vi "bats.parser.hostToFpga.testRunner.vi"(9 "Test.Messages":variant[](array[variant]), 10 "Expected OrderBook.Command[]":T1[](array[typedef])=[{"type"=enum."AddOrder", "side"=66, "orderId "=3544385890602799695, "quantity"=20000, "symbol"=4702127773838213120, "price"=9050, "executed.qty"=0, "canceled.qty"=0, "remaining.qty"=0, "seconds"=0, "nanoseconds"=447000, "Add"=FALSE, "Edit"=FALSE, "Remove"=FALSE}, {"type"=enum."AddOrder", "side"=67, "orderId "=0, "quantity"=30000, "symbol"=4702127773838213120, "price"=9060, "executed.qty"=0, "canceled.qty"=0, "remaining.qty"=0, "seconds"=0, "nanoseconds"=447000, "Add"=FALSE, "Edit"=FALSE, "Remove"=FALSE}] {"symbol" format="%.0x"; "orderId" format="%.0x"; "side" format="%.0x"}, 11 "Test.MessagesOld":T3[](array[typedef])) -> (0 "Failures.Count":i32=1, 2 "Passed":bool, 3 "OrderBook.Command[]":T1[](array[typedef]) {"symbol" format="%.0x"; "orderId" format="%.0x"; "side" format="%.0x"}, 4 "Debug":u64[](array[numeric]) format="%.0x")   [LabVIEW 2022 SP3]
uses:
  fpga/common/orderbook.command.ctl
  fpga/common/orderbook.command.type.ctl
  Message.Spec.ctl
  pitch/oldMessageType.ctl
  pitch/AddOrder/AddOrderLong.Parameters.ctl
  pitch/Time/Time.Parameters.ctl
  pitch/SequencedUnitHeader/SequencedUnitHeader.Parameters.ctl
  pitch/ModifyOrder/ModifyOrderLong.Parameters.ctl
  <vilib>/rvi/interface/RandomDataEmulation/nirviRandomDataOpen.vi
  <vilib>/rvi/interface/common/niFpgaCacheSessionInfoDynamic.vi
  <vilib>/Utility/error.llb/Error Cluster From Error Code.vi
  <vilib>/rvi/errors/niLvFpgaAdjustHostInterfaceError.vi
  <vilib>/FPGAPlugInAG/Dynamic/niLvFpga_Close_Dynamic.vi
  <vilib>/rvi/interface/nirviOpenFPGA/nirviOpenFPGA.xnode
  fpga/bats.parser/bats.parser.test.vi
  <vilib>/rvi/interface/nirviReadWriteControl/nirviReadWriteControl.xnode
  <vilib>/rvi/interface/nirviMethod/nirviMethod.xnode
  <vilib>/rvi/interface/nirviCloseFPGA/nirviCloseFPGA.xnode
  <vilib>/rvi/errors/niLvFpgaMergeErrorWithErrorCode.vi
  <vilib>/FPGAPlugInAG/Dynamic/niLvFpga_ReadFifo_Dynamic.vi
  <vilib>/rvi/interface/Simulation/niFpgaSimulationCallBeginRW.vi
  NiFpgaLv.dll
  <vilib>/FPGAPlugInAG/Dynamic/niLvFpga_WriteFifo_Dynamic.vi
  pitch/SequencedUnitHeader/SequencedUnitHeader.lvclass
  pitch/Time/Time.lvclass
  pitch/AddOrder/AddOrderLong.lvclass
  pitch/ModifyOrder/ModifyOrderLong.lvclass
panel:
  out "size(s)":i32
  out "Words.Out":u16[](array[numeric]) format="%.0x"
  out "Data.size":i32=16
  in  "Execute?":bool=TRUE
  out "Data":u64[](array[numeric]) format="%.0x"
  out "error out":errorcluster
  in  "error in":errorcluster
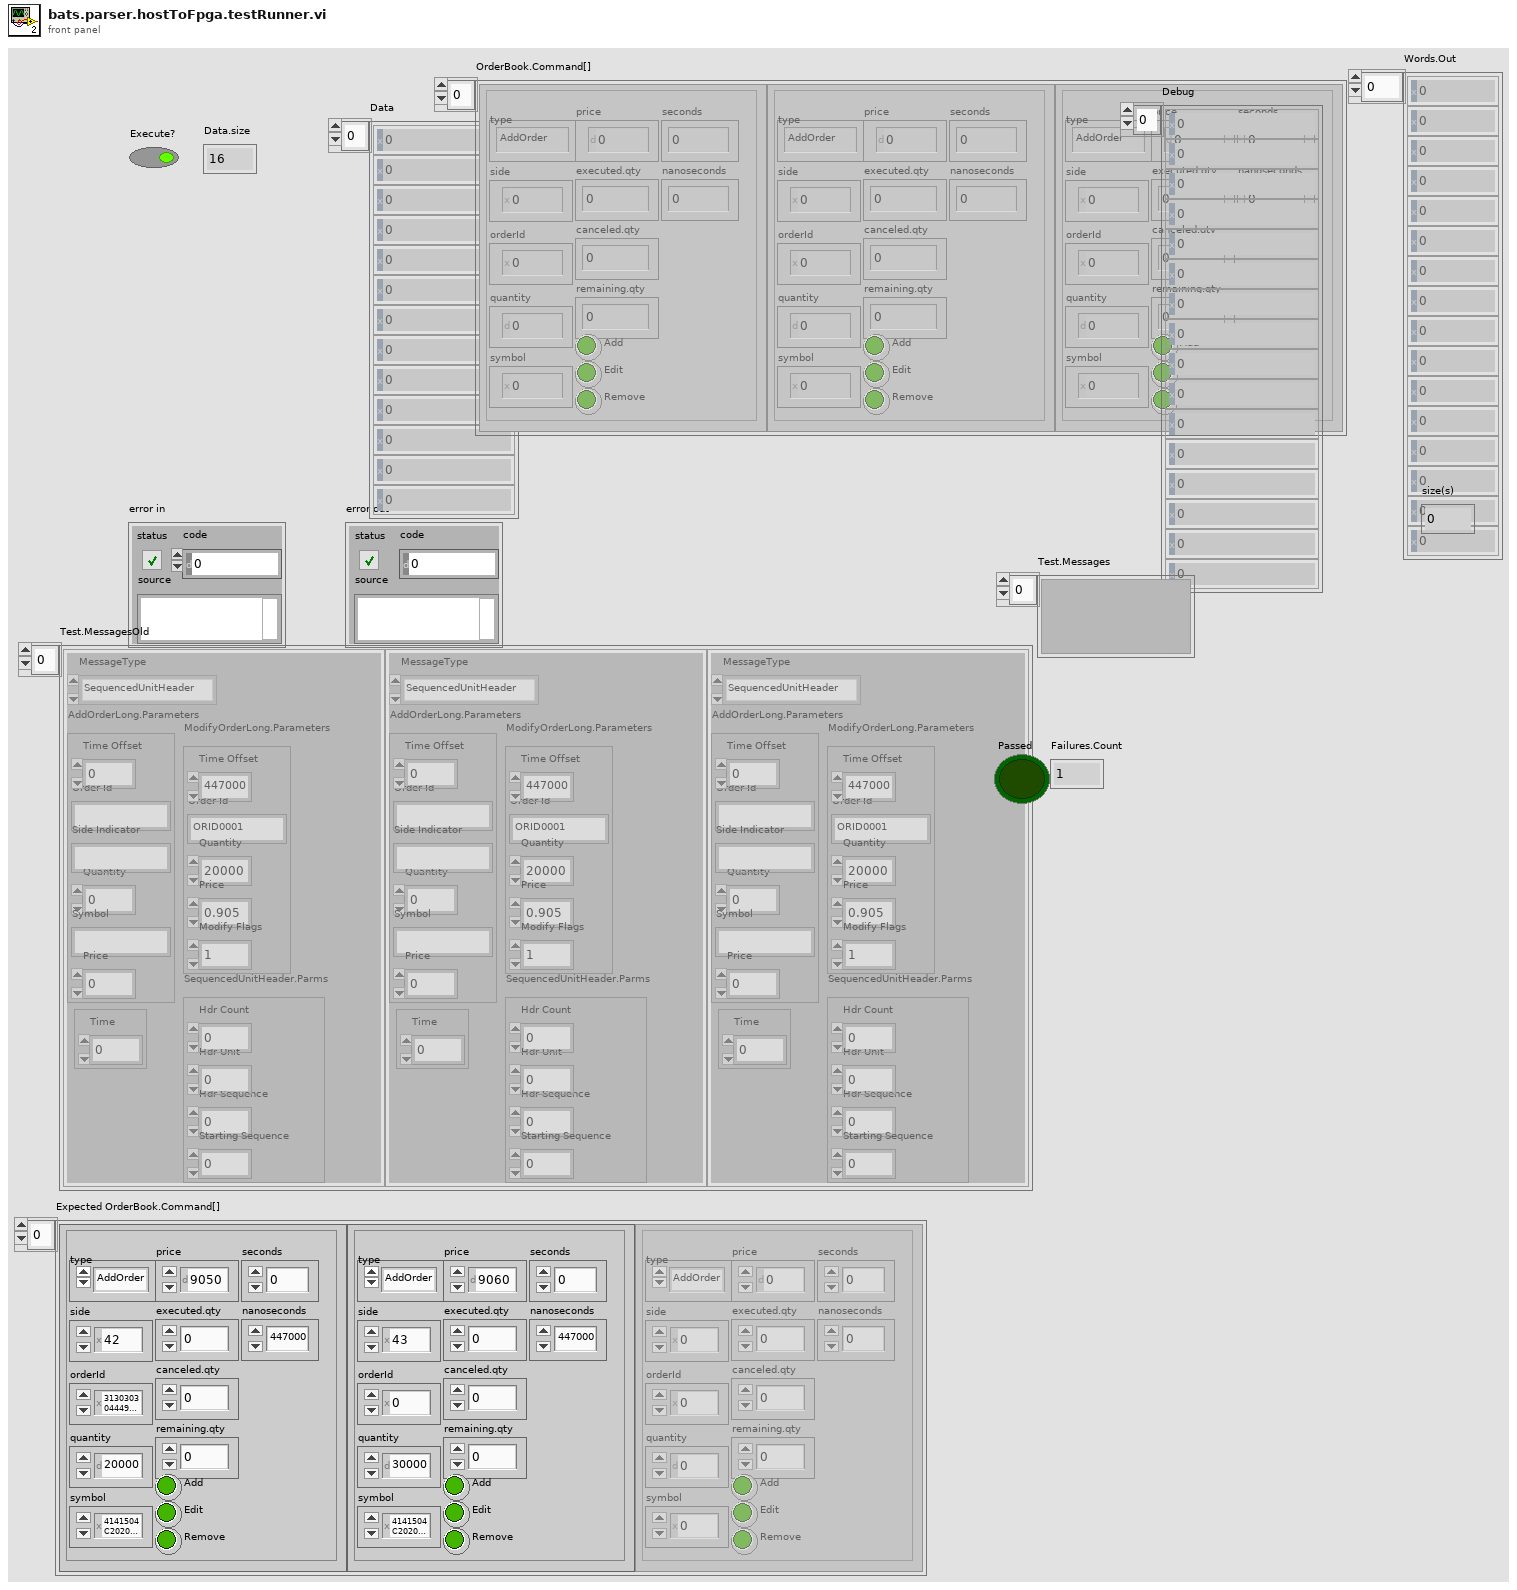
[diagram p1: front panel]
types:
  T1 = typedef "orderbook.command.ctl" = cluster{"type":T2, "side":u8, "orderId ":u64, "quantity":u32, "symbol":u64, "price":u64, "executed.qty":u32, "canceled.qty":u32, "remaining.qty":u32, "seconds":u64, "nanoseconds":u64, "Add":bool, "Edit":bool, "Remove":bool}
  T2 = typedef "orderbook.command.type.ctl" = enum8{"Time", "AddOrder", "OrderExecuted", "OrderExecutedAtPrice", "ReduceSize", "ModifyOrder", "DeleteOrder", "Get.Everything", "Get.All.Orders", "Get.Top"}
  T3 = typedef "Message.Spec.ctl" = cluster{"MessageType":T4, "AddOrderLong.Parameters":T5, "Time.Parms":T6, "SequencedUnitHeader.Parms":T7, "ModifyOrderLong.Parameters":T8}
  T4 = typedef "oldMessageType.ctl" = enum16{"Time", "SequencedUnitHeader", "AddOrderLong", "AddOrderShort", "AddOrderExpanded", "ModifyOrderLong"}
  T5 = typedef "AddOrderLong.lvclass/AddOrderLong.Parameters.ctl" = cluster{"Time Offset":u32, "Order Id":string, "Quantity":u32, "Symbol":string, "Side Indicator":string, "Price":dbl}
  T6 = typedef "Time.lvclass/Time.Parameters.ctl" = cluster{"Time":u32}
  T7 = typedef "SequencedUnitHeader.lvclass/SequencedUnitHeader.Parameters.ctl" = cluster{"Hdr Count":u8, "Hdr Unit":u8, "Hdr Sequence":u32, "Starting Sequence":u32}
  T8 = typedef "ModifyOrderLong.lvclass/ModifyOrderLong.Parameters.ctl" = cluster{"Time Offset":u32, "Order Id":string, "Quantity":u32, "Price":dbl, "Modify Flags":u8}
  T9 = cluster{"type":bool, "side":bool, "orderId ":bool, "quantity":bool, "symbol":bool, "price":bool, "executed.qty":bool, "canceled.qty":bool, "remaining.qty":bool, "seconds":bool, "nanoseconds":bool, "Add":bool, "Edit":bool, "Remove":bool}
  T10 = cluster{"Index":i32, "x = y?":cluster{"type":bool, "side":bool, "orderId ":bool, "quantity":bool, "symbol":bool, "price":bool, "executed.qty":bool, "canceled.qty":bool, "remaining.qty":bool, "seconds":bool, "nanoseconds":bool, "Add":bool, "Edit":bool, "Remove":bool}}
  T11 = cluster{"Index":i32, "x = y?":cluster{"type":bool, "side":bool, "orderId ":bool, "quantity":bool, "symbol":bool, "price":bool, "executed.qty":bool, "canceled.qty":bool, "remaining.qty":bool, "seconds":bool, "nanoseconds":bool, "Add":bool, "Edit":bool, "Remove":bool}}[]
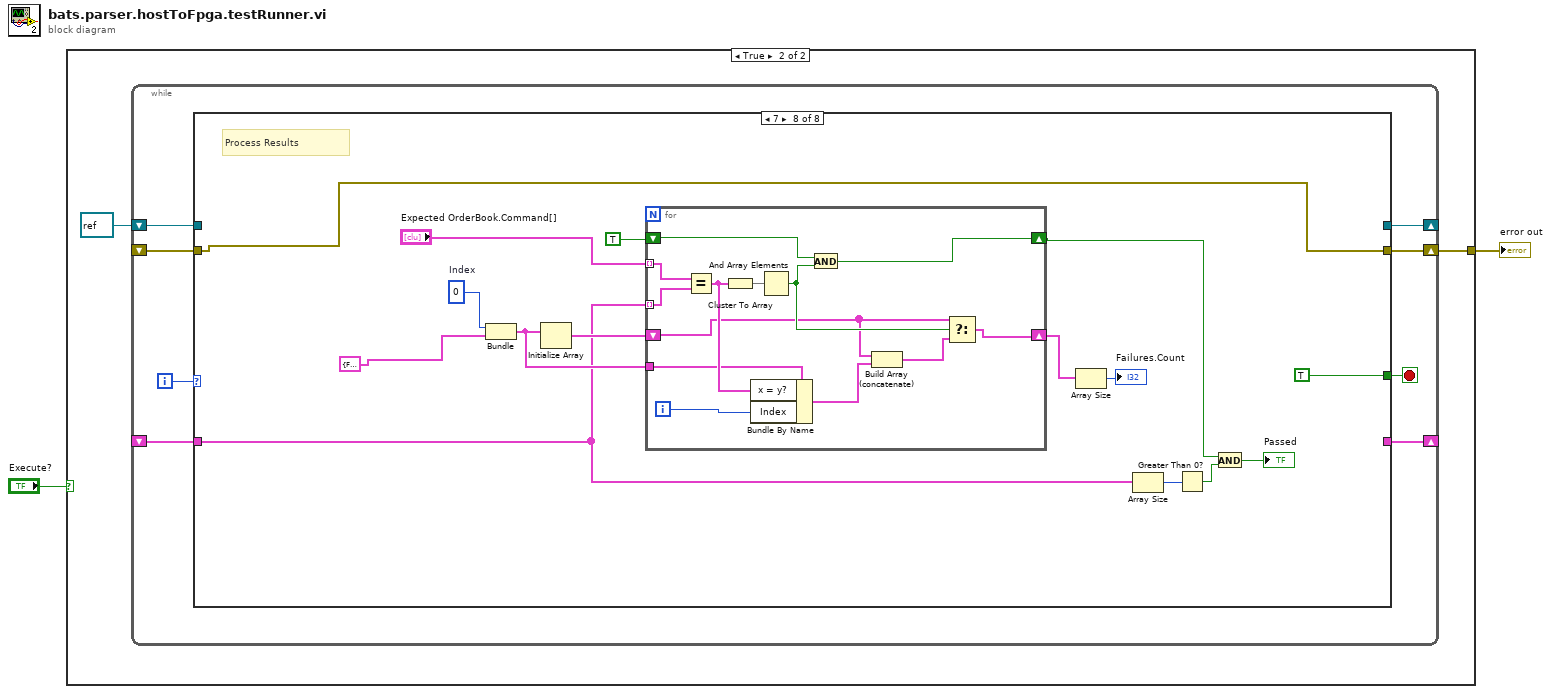
[diagram p0: block diagram]
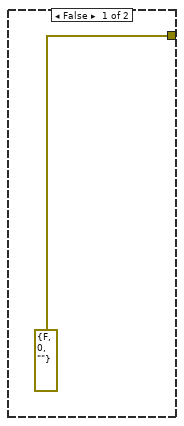
[diagram p2: hidden frame]
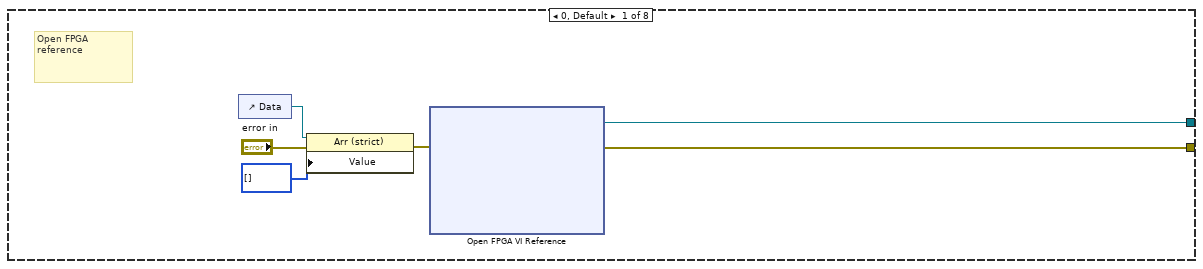
[diagram p3: hidden frame]
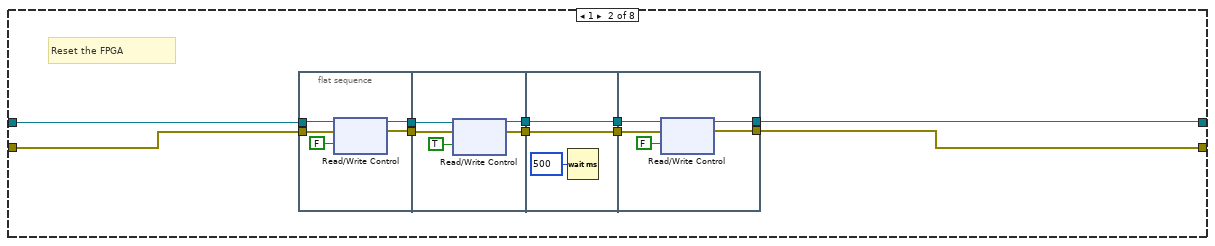
[diagram p4: hidden frame]
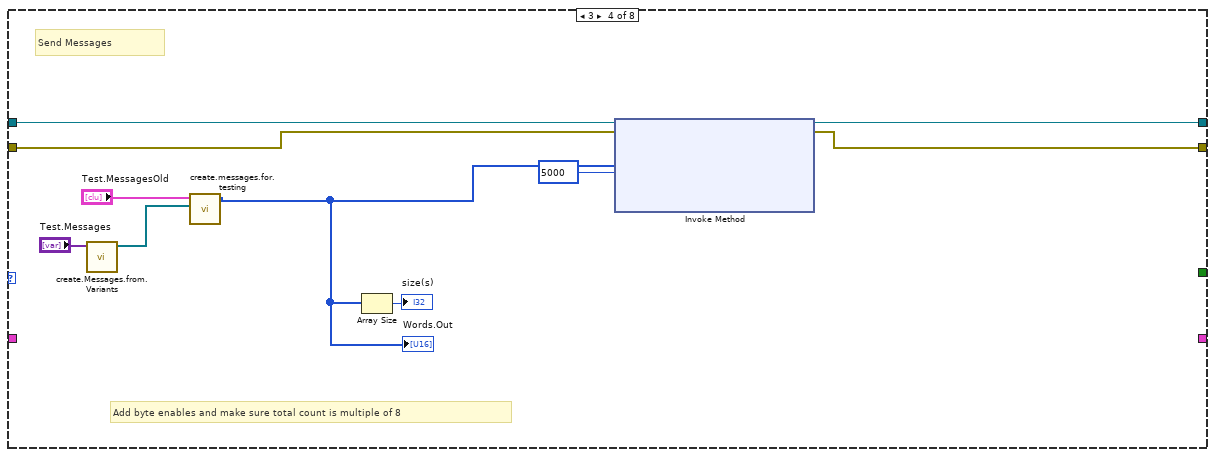
[diagram p6: hidden frame]
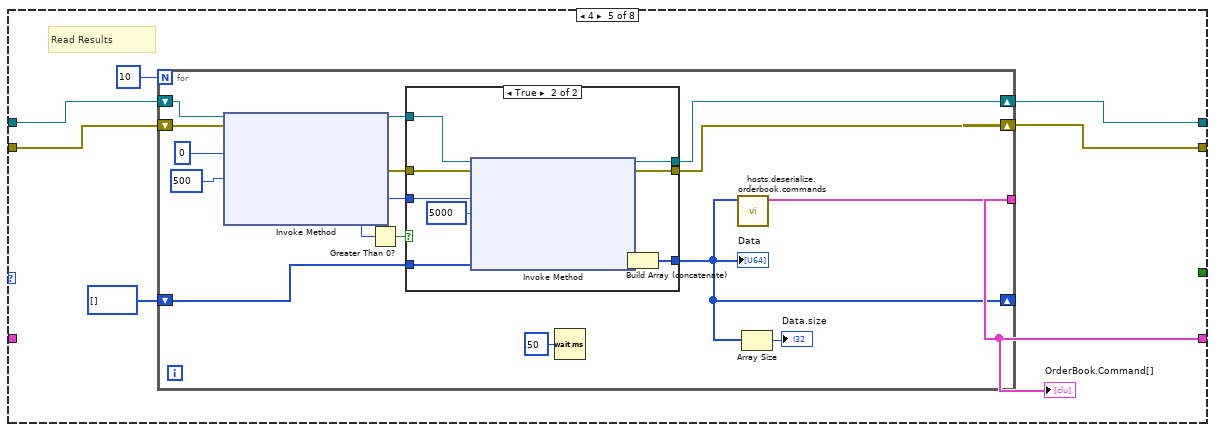
[diagram p7: hidden frame]
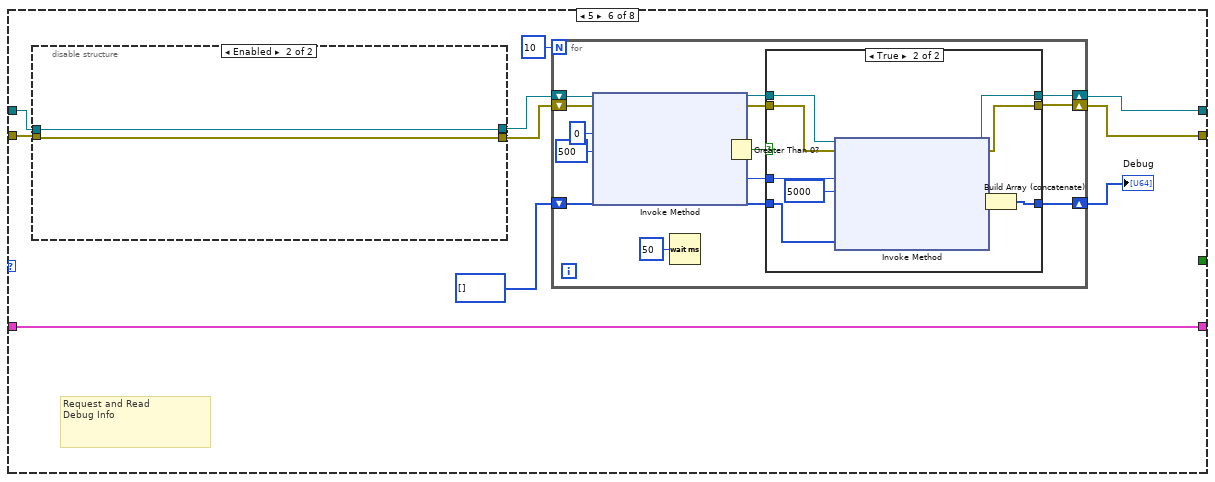
[diagram p9: hidden frame]
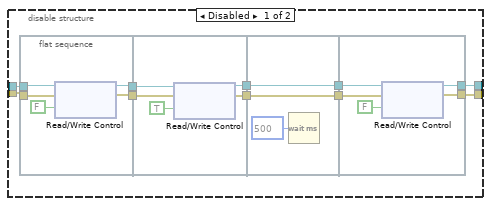
[diagram p10: hidden frame]
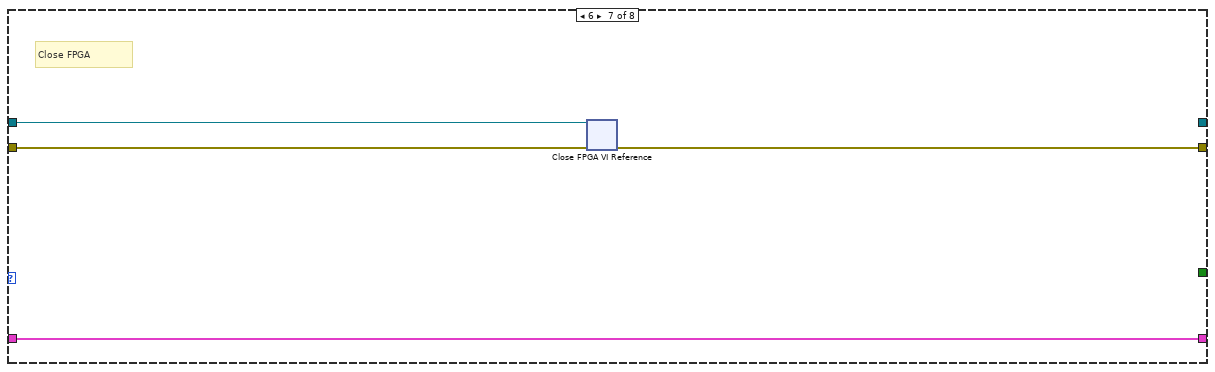
[diagram p12: hidden frame]
diagram:
  n1 = case shown="True" "Execute?" {
    tunnel: [errorcluster {"status"=FALSE, "code"=0, "source"=""} ("error out") w5] -> w2
    frame False {
    }
    frame True {
      n2 = while {
        shift-right: [w11] -> _
        shift-left: refnum<k20> refnum ("FPGA VI Reference Out") -> [w9]
        shift-right: [w10] -> w5
        shift-left: _ -> [w8]
        shift-right: [w7] -> _
        shift-left: _ -> [w6]
        i -> [w13]
        stop <- w12 stop-if-true
        n3 = case shown="7" w13 {
          tunnel: [_ _ _ _ _ _ _ TRUE] -> w12
          tunnel: [w14 w20 w49 w55 w61 w98 _ _] -> w11
          tunnel: [w15 w21 w48 w54 w62 w99 w162 w164] -> w10
          tunnel: w9 -> [_ w23 w49 w57 w64 w102 w161 _]
          tunnel: w8 -> [_ w22 w48 w56 w63 w103 w160 w164]
          tunnel: [_ _ _ _ w60 w94 w159 _] -> w7
          tunnel: w6 -> [_ _ _ _ _ w94 w159 w165]
          frame 0, Default {
            # "Open FPGA\nreference"
            n4 = control-ref of="Data"() -> (w17:refnum<vi>)
            n5 = property class="Arr (strict)"(reference=w17, error in="error in", "Value"=u8[] []) -> (error out=w19:errorcluster)  [unwired: 1 out]
            n6 = xnode ("Open FPGA VI Reference")("error in"=w19) -> ("FPGA VI Reference Out"=w14:refnum<k20>, "error out"=w15:errorcluster)  [unwired: 1 in]
          }
          frame 1 {
            # "Reset the FPGA"
            n7 = flat-sequence {
              tunnel: w23 -> [w31]
              tunnel: w22 -> [w32]
              tunnel: [w33] -> w29
              tunnel: [w34] -> w28
              tunnel: [w38] -> w27
              tunnel: [w37] -> w26
              tunnel: w29 -> [w36]
              tunnel: w28 -> [w35]
              tunnel: [w42] -> w25
              tunnel: w27 -> [w42]
              tunnel: w26 -> [w41]
              tunnel: [w41] -> w24
              tunnel: w25 -> [w46]
              tunnel: w24 -> [w45]
              tunnel: [w44] -> w21
              tunnel: [w43] -> w20
              frame #0 {
                n8 = xnode "Read/Write Control"("FPGA VI Reference In"=w31, "error in"=w32, "reset"=FALSE) -> ("FPGA VI Reference Out"=w34:refnum<k20>, "error out"=w33:errorcluster)
              }
              frame #1 {
                n9 = xnode "Read/Write Control"("FPGA VI Reference In"=w35, "error in"=w36, "reset"=TRUE) -> ("FPGA VI Reference Out"=w37:refnum<k20>, "error out"=w38:errorcluster)
              }
              frame #2 {
                n10 = Wait (ms)(milliseconds to wait=u32 500) -> ()  [unwired: 1 out]
              }
              frame #3 {
                n11 = xnode "Read/Write Control"("FPGA VI Reference In"=w45, "error in"=w46, "reset"=FALSE) -> ("FPGA VI Reference Out"=w43:refnum<k20>, "error out"=w44:errorcluster)
              }
            }
          }
          frame 2 {
            # "Memory Configuration"
          }
          frame 3 {
            # "Add byte enables and make sure total count is multiple of 8"
            # "Send Messages"
            n12 = call "create.Messages.from.Variants.vi"("Messages.Variant"="Test.Messages") -> ("Messages"=w50:refnum<class "MessageBase.lvclass">[])  [unwired: 10 in]
            n13 = call "create.messages.for.testing.vi"("Message.to.Create"=w50, "Messages to Create"="Test.MessagesOld") -> ("Words.Out"=w53:u16[])  [unwired: 9 in]
            "Words.Out" <- w53
            n14 = Array Size(array=w53) -> (size(s)=→"size(s)":i32)
            n15 = xnode "Invoke Method"("FPGA VI Reference In"=w57, "error in"=w56, "Data"=w53, "Timeout (ms)"=5000) -> ("FPGA VI Reference Out"=w55:refnum<k20>, "error out"=w54:errorcluster)  [unwired: 1 out]
          }
          frame 4 {
            # "Read Results"
            n16 = for {
              N: 10 -> [_]
              shift-right: [w69] -> _
              shift-left: u64[] [] -> [w74]
              shift-right: [w73] -> w61
              shift-left: w64 -> [w81]
              shift-right: [w72] -> w62
              shift-left: w63 -> [w80]
              tunnel: [w67] -> w60
              n17 = xnode "Invoke Method"("FPGA VI Reference In"=w81, "error in"=w80, "Number of Elements"=u32 0, "Timeout (ms)"=500) -> ("FPGA VI Reference Out"=w75:refnum<k20>, "error out"=w71:errorcluster, "Elements Remaining"=w76:u32)  [unwired: 1 out]
              n18 = Greater Than 0?(x=w76) -> (x > 0?=w77:bool)
              n19 = case shown="True" w77 {
                tunnel: w76 -> [_ w93]
                tunnel: w75 -> [w83 w91]
                tunnel: [w84 w88] -> w69
                tunnel: w74 -> [w84 w90]
                tunnel: [w83 w87] -> w73
                tunnel: [w82 w86] -> w72
                tunnel: w71 -> [w82 w85]
                frame False {
                }
                frame True {
                  n20 = xnode "Invoke Method"("FPGA VI Reference In"=w91, "error in"=w85, "Number of Elements"=w93, "Timeout (ms)"=5000) -> ("FPGA VI Reference Out"=w87:refnum<k20>, "error out"=w86:errorcluster, "Data"=w89:u64[])  [unwired: 1 out]
                  n21 = Build Array (concatenate)(w90, w89) -> (w88:u64[])
                }
              }
              "Data" <- w69
              n22 = Wait (ms)(milliseconds to wait=u32 50) -> ()  [unwired: 1 out]
              n23 = call "hosts.deserialize.orderbook.commands.vi"("DataIn"=w69) -> ("OrderBook.Command[]"=w67:T1[])  [unwired: 10 in]
              n24 = Array Size(array=w69) -> (size(s)=→"Data.size":i32)
            }
            "OrderBook.Command[]" <- w60
          }
          frame 5 {
            # "Request and Read\nDebug Info"
            n25 = disable-structure shown="Enabled" {
              disable-tunnel: w103 -> [w107 w132]
              disable-tunnel: w102 -> [w106 w133]
              disable-tunnel: [w105 w133] -> w101
              disable-tunnel: [w104 w132] -> w100
              frame Disabled {
                n26 = flat-sequence {
                  tunnel: w106 -> [w115]
                  tunnel: w107 -> [w116]
                  tunnel: [w117] -> w113
                  tunnel: [w118] -> w112
                  tunnel: [w122] -> w111
                  tunnel: [w121] -> w110
                  tunnel: w113 -> [w120]
                  tunnel: w112 -> [w119]
                  tunnel: [w126] -> w109
                  tunnel: w111 -> [w126]
                  tunnel: w110 -> [w125]
                  tunnel: [w125] -> w108
                  tunnel: w109 -> [w130]
                  tunnel: w108 -> [w129]
                  tunnel: [w128] -> w104
                  tunnel: [w127] -> w105
                  frame #0 {
                    n27 = xnode "Read/Write Control"("FPGA VI Reference In"=w115, "error in"=w116, "debug"=FALSE ("reset")) -> ("FPGA VI Reference Out"=w118:refnum<k20>, "error out"=w117:errorcluster)
                  }
                  frame #1 {
                    n28 = xnode "Read/Write Control"("FPGA VI Reference In"=w119, "error in"=w120, "debug"=TRUE ("reset")) -> ("FPGA VI Reference Out"=w121:refnum<k20>, "error out"=w122:errorcluster)
                  }
                  frame #2 {
                    n29 = Wait (ms)(milliseconds to wait=u32 500) -> ()  [unwired: 1 out]
                  }
                  frame #3 {
                    n30 = xnode "Read/Write Control"("FPGA VI Reference In"=w129, "error in"=w130, "debug"=FALSE ("reset")) -> ("FPGA VI Reference Out"=w127:refnum<k20>, "error out"=w128:errorcluster)
                  }
                }
              }
              frame Enabled {
              }
            }
            n31 = for {
              N: 10 -> [_]
              shift-right: [w140] -> w98
              shift-left: w101 -> [w146]
              shift-right: [w139] -> w99
              shift-left: w100 -> [w145]
              shift-right: [w141] -> w97
              shift-left: u64[] [] -> [w135]
              n32 = xnode "Invoke Method"("FPGA VI Reference In"=w146, "error in"=w145, "Number of Elements"=u32 0, "Timeout (ms)"=500) -> ("FPGA VI Reference Out"=w138:refnum<k20>, "error out"=w137:errorcluster, "Elements Remaining"=w136:u32)  [unwired: 1 out]
              n33 = Wait (ms)(milliseconds to wait=u32 50) -> ()  [unwired: 1 out]
              n34 = Greater Than 0?(x=w136) -> (x > 0?=w142:bool)
              n35 = case shown="True" w142 {
                tunnel: [w147 w157] -> w141
                tunnel: [w149 w156] -> w140
                tunnel: [w148 w155] -> w139
                tunnel: w138 -> [w149 w154]
                tunnel: w137 -> [w148 w153]
                tunnel: w136 -> [_ w152]
                tunnel: w135 -> [w147 w150]
                frame False {
                }
                frame True {
                  n36 = xnode "Invoke Method"("FPGA VI Reference In"=w154, "error in"=w153, "Number of Elements"=w152, "Timeout (ms)"=5000) -> ("FPGA VI Reference Out"=w156:refnum<k20>, "error out"=w155:errorcluster, "Data"=w158:u64[])  [unwired: 1 out]
                  n37 = Build Array (concatenate)(w150, w158) -> (w157:u64[])
                }
              }
            }
            "Debug" <- w97
          }
          frame 6 {
            # "Close FPGA"
            n38 = xnode "Close FPGA VI Reference"("FPGA VI Reference In"=w161, "error in"=w160) -> ("error out"=w162:errorcluster)
          }
          frame 7 {
            w167 = 0  # Index
            # "Process Results"
            n39 = Bundle("Index"=w167, "x = y?"=T9 {"type"=FALSE, "side"=FALSE, "orderId "=FALSE, "quantity"=FALSE, "symbol"=FALSE, "price"=FALSE, "executed.qty"=FALSE, "canceled.qty"=FALSE, "remaining.qty"=FALSE, "seconds"=FALSE, "nanoseconds"=FALSE, "Add"=FALSE, "Edit"=FALSE, "Remove"=FALSE}) -> (w169:T10)  [unwired: 1 in]
            n40 = Initialize Array(w169) -> (w168:T11)  [unwired: 1 in]
            n41 = for {
              tunnel: "Expected OrderBook.Command[]" -> [w190] mode=indexing
              tunnel: w165 -> [w189] mode=indexing
              shift-right: [w187] -> w176
              shift-left: TRUE -> [w188]
              shift-right: [w184] -> w170
              shift-left: w168 -> [w179]
              tunnel: w169 -> [w182]
              i -> [w181]
              n42 = Equal?(x=w190, y=w189) -> (x = y?=w183:T9)
              n43 = Cluster To Array(cluster=w183) -> (array=w186:bool[])
              n44 = Bundle By Name(cluster=w182, "x = y?"=w183, "Index"=w181) -> (w180:T10)
              n45 = And Array Elements(Boolean array=w186) -> (logical AND=w185:bool)
              n46 = And(x=w188, y=w185) -> (x .and. y?=w187:bool)
              n47 = Build Array (concatenate)(w179, w180) -> (w178:T11)
              n48 = Select(t=w179, s=w185, f=w178) -> (s? t:f=w184:T11)
            }
            n49 = Array Size(array=w170) -> (size(s)=→"Failures.Count":i32)
            n50 = Array Size(array=w165) -> (size(s)=w173:i32)
            n51 = Greater Than 0?(x=w173) -> (x > 0?=w174:bool)
            n52 = And(x=w176, y=w174) -> (x .and. y?=→"Passed":bool)
          }
        }
      }
    }
  }
  "error out" <- w2
